vi "LoopAndQueryInput.vi"(3 "error in":errorcluster, 4 "Input channel selection":T1, 5 "VISA Refnum in":refnum<visa-resource-name>) -> (0 "error out":errorcluster, 1 "Error signal / V":dbl[](array[numeric]), 2 "VISA resource name out":refnum<visa-resource-name>)   [LabVIEW 2015]
doc: "Loop through a selection of input channels and query the device for each one that is selected"
uses:
  controls/ChannelSelection.ctl
  Driver/Typedefs/InputChannelTypedef.ctl
  Driver/YbTempCtrl.lvlib
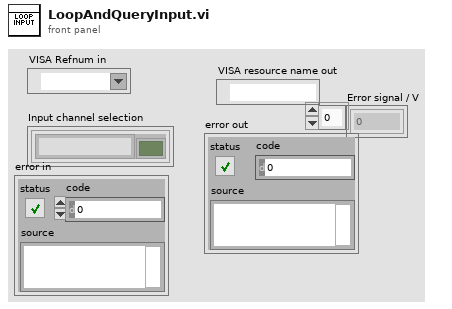
[diagram p1: front panel]
types:
  T1 = typedef "ChannelSelection.ctl" = cluster{"Channel name":string, "Enum id":u16, "Logging?":bool}[]
  T2 = typedef "YbTempCtrl.lvlib/InputChannelTypedef.ctl" = enum16{"1T", "2T", "TMP", "POW"}
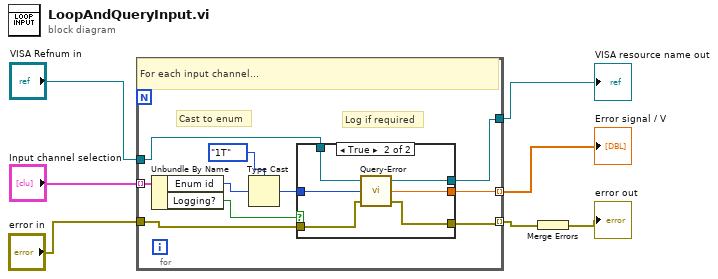
[diagram p0: block diagram]
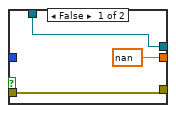
[diagram p2: hidden frame]
diagram:
  n1 = for {
    tunnel: "Input channel selection" -> [w16] mode=indexing
    tunnel: "VISA Refnum in" -> [w12]
    tunnel: [w9] -> w7 mode=indexing
    tunnel: [w8] -> w3
    tunnel: "error in" -> [w10]
    tunnel: [w11] -> w1 mode=indexing
    # "Log if required"
    # "Cast to enum"
    # "For each input channel..."
    n2 = Unbundle By Name(w16) -> ("Enum id"=w15:u16, "Logging?"=w14:bool)
    n3 = Type Cast(type=InputChannelTypedef."1T" ("Input channel"), x=w15) -> (*(type *) &x=w13:T2)
    n4 = case shown="True" w14 {
      tunnel: w13 -> [_ w26]
      tunnel: w12 -> [w18 w25]
      tunnel: w10 -> [w19 w24]
      tunnel: [w19 w23] -> w11
      tunnel: [nan ("Error Signal / V") w22] -> w9
      tunnel: [w18 w21] -> w8
      frame False {
      }
      frame True {
        n5 = call "Query-Error.vi"("error in (no error)"=w24, "Input channel"=w26, "VISA resource name"=w25) -> ("error out"=w23:errorcluster, "Error Signal / V"=w22:dbl, "VISA resource name out"=w21:refnum<visa-resource-name>)
      }
    }
  }
  "Error signal / V" <- w7
  "VISA resource name out" <- w3
  n6 = Merge Errors(w1) -> (→"error out":errorcluster)
